vi "Cleanup.vi"(8 "error in (no error)":errorcluster, 11 "Websocket Client in":refnum<class "Websocket Client.lvclass">) -> (0 "error out":errorcluster)   [LabVIEW 2020, in "Stream-Websocket.lvlib" / "Websocket Client.lvclass"]
uses:
  Websocket Client.lvclass
  Websocket Client.lvclass/Websocket Client.ctl
  <vilib>/IlluminatedG/lv-stream/Connection/Connection.lvclass
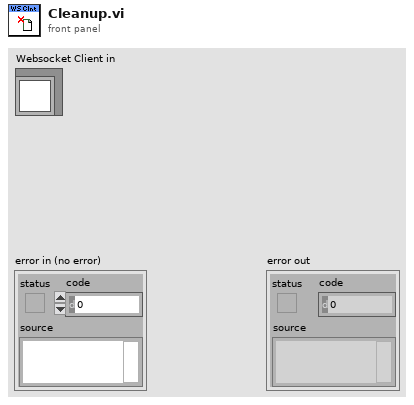
[diagram p1: front panel]
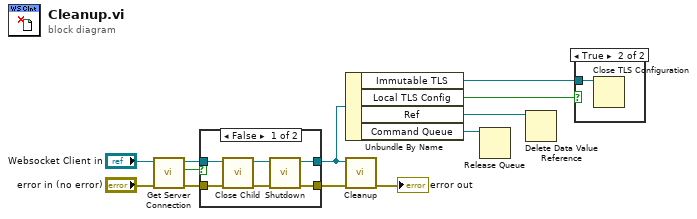
[diagram p0: block diagram]
diagram:
  n1 = call "Get Server Connection.vi"("error in (no error)"="error in (no error)", "Websocket Client in"="Websocket Client in") -> ("error out"=w7:errorcluster, "Server Connection"=w9:bool, "Websocket Client out"=w8:refnum<class "Websocket Client.lvclass">)  [unwired: 7 in]
  n2 = case shown="False" w9 {
    tunnel: w8 -> [w18 w20]
    tunnel: w7 -> [w17 w19]
    tunnel: [w13 w20] -> w5
    tunnel: [w14 w19] -> w6
    frame False {
      n3 = call-dynamic "Close Child.vi"("error in (no error)"=w17, "Websocket Client in"=w18) -> ("error out"=w15:errorcluster, "Websocket Client out"=w16:refnum<class "Websocket Client.lvclass">)  [unwired: 8 in]
      n4 = call "Shutdown.vi"("error in (no error)"=w15, "Websocket Client in"=w16) -> ("error out"=w14:errorcluster, "Websocket Client out"=w13:refnum<class "Websocket Client.lvclass">)  [unwired: 8 in]
    }
    frame True {
    }
  }
  n5 = Unbundle By Name(w5) -> ("Immutable TLS"=w1:refnum<k36>, "Local TLS Config"=w2:bool, "Ref"=w3:refnum<data-value>, "Command Queue"=w4:refnum<queue>)
  n6 = call-parent "Cleanup.vi"("error in (no error)"=w6, "Connection in"=w5) -> ("error out"=→"error out":errorcluster)  [unwired: 9 in]
  n7 = Release Queue(queue=w4) -> ()  [unwired: 2 in, 3 out]
  n8 = Delete Data Value Reference(data value reference=w3) -> ()  [unwired: 1 in, 2 out]
  n9 = case shown="True" w2 {
    tunnel: w1 -> [_ w21]
    frame False {
    }
    frame True {
      n10 = Close TLS Configuration(11:w21) -> ()  [unwired: 1 in, 1 out]
    }
  }
